vi "Set Sensor Glue Gap.vi"() -> ()   [LabVIEW 2016]
uses:
  Classes/Controller/Controller.lvclass
  Classes/Workspace/Fixture.lvclass
  Classes/Workspace/Fixture Enum.ctl
  Classes/Routine/Routine Enum.ctl
  Classes/Routine/Routine.lvclass
  Classes/Routine/Pick and Place/Pick and Place.lvclass
  Classes/Controller/Motion/Motion.lvclass
  Classes/Controller/I-O/I-O.lvclass
panel:
  in  "Tool Height":dbl
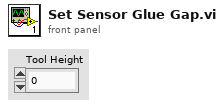
[diagram p1: front panel]
types:
  T1 = typedef "Fixture.lvclass/Fixture Enum.ctl" = enum16{"Assembly Tray", "Syringe Space", "Component", "Pick Up Tool", "Current Position"}
  T2 = typedef "Routine.lvclass/Routine Enum.ctl" = enum16{"Primary Pick Up", "Pick Up All", "Put Down Secondary", "Put Down All", "Release Syringe", "Secondary Pick Up", "Secure Syringe", "Dispense on Plate", "Dispense on Kapton", "Dispense on Sensor"}
  T3 = typedef "Controller.lvclass/Controllers.ctl" = cluster{"I-O.lvclass":refnum<class "I-O.lvclass">, "Motion.lvclass":refnum<class "Motion.lvclass">, "Dispenser.lvclass":refnum<class "Dispenser.lvclass">}
  T4 = typedef "Fixture.lvclass/Workspace.ctl" = cluster{"XYZTheta":dbl[], "Workspace Valve":i32, "Workspace Sensor":i32}
  T5 = typedef "I-O.lvclass/Pin Map.ctl" = cluster{"Region Valves":i32[], "Extra Valves":dbl[][][], "Tool Primary Valve":i32, "Tool Secondary Valve":i32, "Region Sensors":i32[], "Extra Sensors":dbl[][][], "Tool Primary Sensor":dbl, "Tool Secondary Sensor":dbl, "Compression Sensor":dbl, "5V":i32}
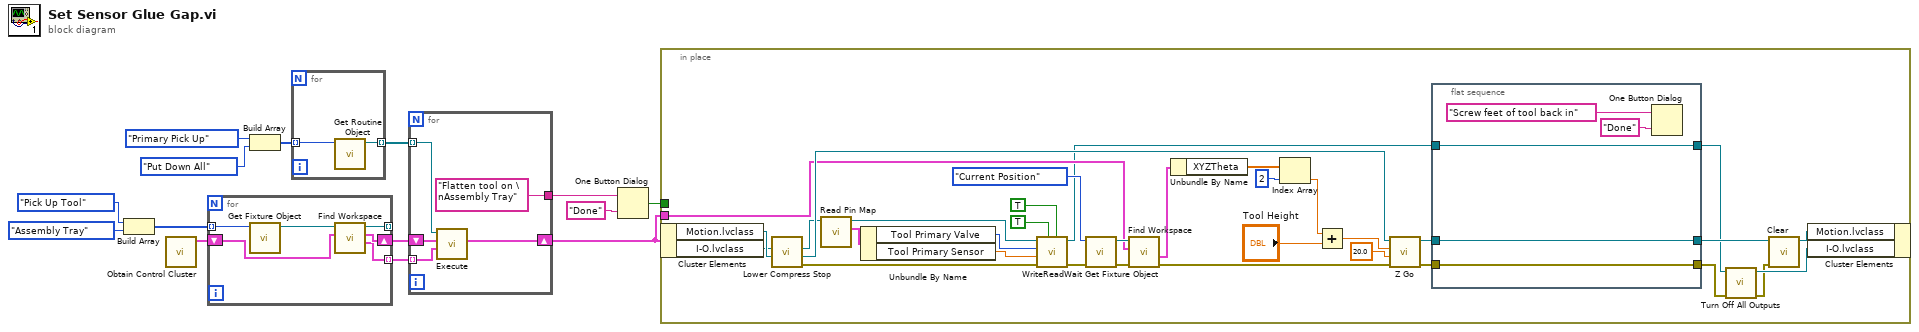
[diagram p0: block diagram]
diagram:
  n1 = Build Array(Fixture_Enum."Pick Up Tool" ("Fixture"), Fixture_Enum."Assembly Tray" ("Fixture")) -> (w5:T1[])
  n2 = call "Obtain Control Cluster.vi"() -> ("Control Out"=w4:T3)  [unwired: 11 in]
  n3 = for {
    tunnel: w5 -> [w20] mode=indexing
    tunnel: [w19] -> _ mode=indexing
    shift-right: [w17] -> w3
    shift-left: w4 -> [w18]
    tunnel: [w16] -> w2 mode=indexing
    n4 = call "Get Fixture Object.vi"("Fixture"=w20) -> ("Workspace.lvclass"=w15:refnum<class "Fixture.lvclass">)  [unwired: 8 in, 2 out]
    n5 = call-dynamic "Find Workspace.vi"("Control In"=w18, "Workspace In"=w15) -> (1:"Workspace Out"=w16:T4, "Control Out"=w17:T3, 3:"Workspace Out"=w19:refnum<class "Fixture.lvclass">)  [unwired: 6 in, 1 out]
  }
  n6 = Build Array(Routine_Enum."Primary Pick Up" ("Routine"), Routine_Enum."Put Down All" ("Routine")) -> (w12:T2[])
  n7 = for {
    tunnel: w12 -> [w22] mode=indexing
    tunnel: [w21] -> w11 mode=indexing
    n8 = call "Get Routine Object.vi"("Routine"=w22) -> ("Routine out"=w21:refnum<class "Routine.lvclass">)  [unwired: 9 in, 1 out]
  }
  n9 = for {
    shift-right: [w25] -> w1
    shift-left: w3 -> [w26]
    tunnel: w11 -> [w27] mode=indexing
    tunnel: ["Flatten tool on \nAssembly Tray"] -> w10
    tunnel: w2 -> [w23] mode=indexing
    n10 = call-dynamic "Execute.vi"("Workspace"=w23, "Control In"=w26, "Routine in"=w27) -> ("Control Out"=w25:T3)  [unwired: 6 in, 2 out]
  }
  n11 = One Button Dialog(message=w10, button name ("OK")="Done") -> (true=w8:bool)
  n12 = in-place {
    in-place-border: w8 -> [_]
    in-place-border: w1 -> [w45]
    n13 = in-place-cluster #1(w1) -> ("Motion.lvclass"=w49:refnum<class "Motion.lvclass">, "I-O.lvclass"=w48:refnum<class "I-O.lvclass">)
    n14 = call "Lower Compress Stop.vi"("Motion.lvclass"=w49, "I-O.lvclass"=w48) -> ("error out"=w32:errorcluster, "Motion.lvclass"=w60:refnum<class "Motion.lvclass">, "I-O out"=w38:refnum<class "I-O.lvclass">)  [unwired: 6 in, 1 out]
    n15 = call-dynamic "Read Pin Map.vi"("I-O in"=w38) -> ("Pin Map 2"=w37:T5, "I-O out"=w30:refnum<class "I-O.lvclass">)  [unwired: 8 in, 1 out]
    n16 = Unbundle By Name(w37) -> ("Tool Primary Valve"=w36:i32, "Tool Primary Sensor"=w35:dbl)
    n17 = call "WriteReadWait.vi"("Read Value"=TRUE, "Write Value"=TRUE, "error in (no error)"=w32, "Read"=w35, "Write"=w36, "I-O in"=w30) -> ("error out"=w31:errorcluster, "I-O out"=w29:refnum<class "I-O.lvclass">)  [unwired: 4 in]
    n18 = call "Get Fixture Object.vi"("error in (no error)"=w31, "Fixture"=Fixture_Enum."Current Position") -> ("error out"=w40:errorcluster, "Workspace.lvclass"=w46:refnum<class "Fixture.lvclass">)  [unwired: 7 in, 1 out]
    n19 = call-dynamic "Find Workspace.vi"("Error In"=w40, "Control In"=w45, "Workspace In"=w46) -> ("Error Out"=w39:errorcluster, "Workspace Out"=w44:T4)  [unwired: 5 in, 2 out]
    n20 = Unbundle By Name(w44) -> ("XYZTheta"=w43:dbl[])
    n21 = Index Array(array=w43, index=2) -> (element=w41:dbl)
    n22 = Add(x=w41, y="Tool Height") -> (x+y=w59:dbl)
    n23 = call-dynamic "Z Go.vi"("error in (no error)"=w39, "Speed"=20.0 ("Setting Speed"), "Position"=w59, "Motion in"=w60) -> ("error out"=w56:errorcluster, "Motion out"=w57:refnum<class "Motion.lvclass">)  [unwired: 6 in]
    n24 = flat-sequence {
      tunnel: w57 -> [w62]
      tunnel: w56 -> [w64]
      tunnel: [w64] -> w55
      tunnel: [w62] -> w52
      tunnel: w29 -> [w61]
      tunnel: [w61] -> w28
      frame #0 {
        n25 = One Button Dialog(message="Screw feet of tool back in", button name ("OK")="Done") -> ()  [unwired: 1 out]
      }
    }
    n26 = call-dynamic "Turn Off All Outputs.vi"("error in (no error)"=w55, "I-O in"=w28) -> ("error out"=w53:errorcluster, "I-O out"=w54:refnum<class "I-O.lvclass">)  [unwired: 8 in]
    n27 = call "Clear.vi"("error in (no error)"=w53, "Motion in"=w52) -> ("Motion out"=w51:refnum<class "Motion.lvclass">)  [unwired: 8 in, 1 out]
    n28 = in-place-cluster #1("Motion.lvclass"=w51, "I-O.lvclass"=w54) -> ()  [unwired: 1 out]
  }
